vi "MakeSIGMU_Info.vi"(7 "ICM Service in":refnum<class "IcmMessageService.lvclass">, 8 "error in (no error)":errorcluster, 11 "AssetNodes In":T1[](array[typedef])) -> (0 "error out":errorcluster, 3 "SIGMU Output":T6[](array[typedef]))   [LabVIEW 2017]
uses:
  typedefs/Asset Info.ctl
  typedefs/Sensor Info.ctl
  typedefs/Metric Info.ctl
  <vilib>/addons/InsightCM/MessageBus/MessageService/IcmMessageService.lvclass
  <vilib>/addons/InsightCM/MessageBus/Base/controls/AssetNodeView.ctl
  <vilib>/addons/InsightCM/MessageBus/Base/controls/AssetState.ctl
  <vilib>/addons/InsightCM/MessageBus/Base/controls/Metric.ctl
  <vilib>/addons/InsightCM/MessageBus/Base/controls/KeyValuePair.ctl
  <vilib>/addons/InsightCM/MessageBus/Base/controls/AssetNodeReference.ctl
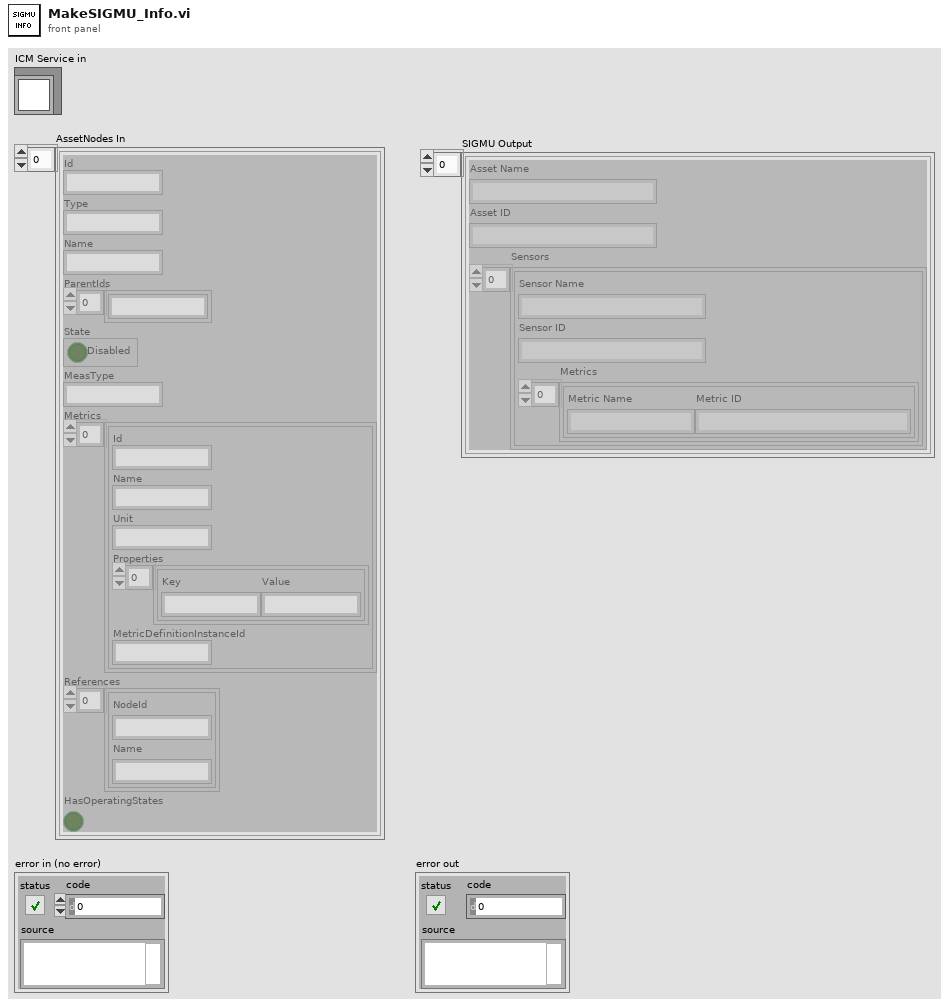
[diagram p1: front panel]
types:
  T1 = typedef "AssetNodeView.ctl" = cluster{"Id":string, "Type":string, "Name":string, "ParentIds":string[], "State":T2, "MeasType":string, "Metrics":T3[], "References":T5[], "HasOperatingStates":bool}
  T2 = typedef "AssetState.ctl" = cluster{"Disabled":bool}
  T3 = typedef "Metric.ctl" = cluster{"Id":string, "Name":string, "Unit":string, "Properties":T4[], "MetricDefinitionInstanceId":string}
  T4 = typedef "KeyValuePair.ctl" = cluster{"Key":string, "Value":string}
  T5 = typedef "AssetNodeReference.ctl" = cluster{"NodeId":string, "Name":string}
  T6 = typedef "Asset Info.ctl" = cluster{"Asset Name":string, "Asset ID":string, "Sensors":T7[]}
  T7 = typedef "Sensor Info.ctl" = cluster{"Sensor Name":string, "Sensor ID":string, "Metrics":T8[]}
  T8 = typedef "Metric Info.ctl" = cluster{"Metric Name ":string, "Metric ID":string}
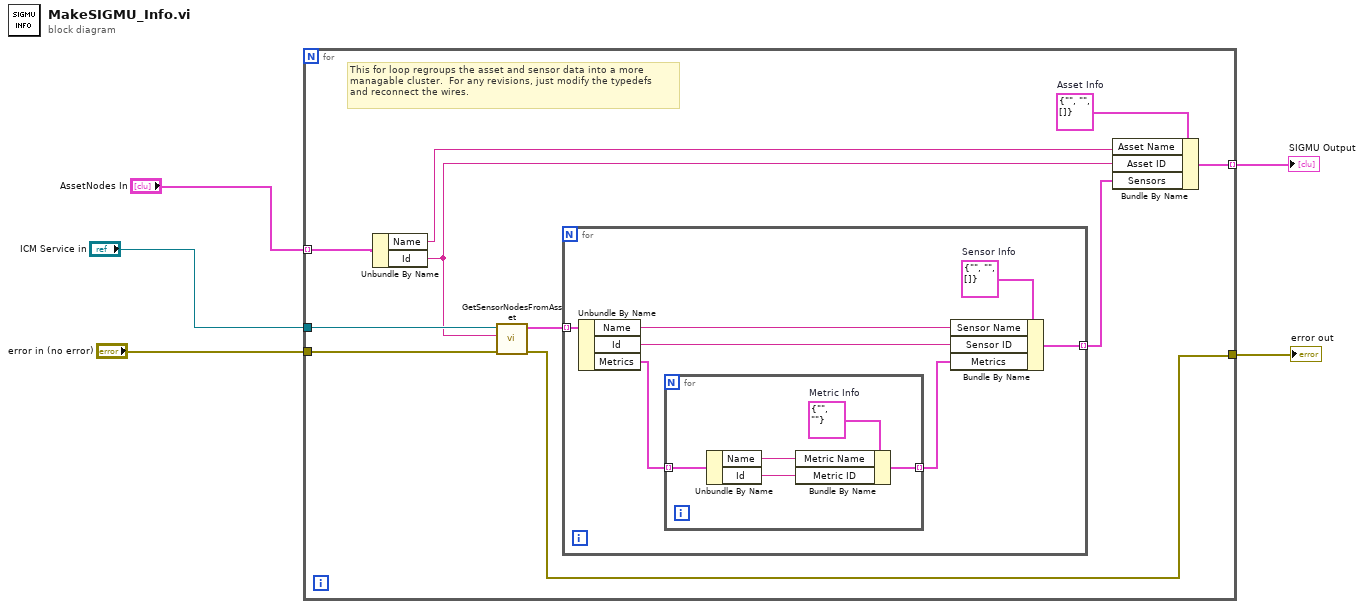
[diagram p0: block diagram]
diagram:
  n1 = for {
    tunnel: "AssetNodes In" -> [w15] mode=indexing
    tunnel: "ICM Service in" -> [w14]
    tunnel: "error in (no error)" -> [w13]
    tunnel: [w7] -> w4 mode=indexing
    tunnel: [w6] -> w5
    w12 = T6 {"Asset Name"="", "Asset ID"="", "Sensors"=[]}  # Asset Info
    # "This for loop regroups the asset and sensor data into a more \nmanagable cluster.  For any revisions, just modify the typedefs\nand reconnect the wires."
    n2 = Unbundle By Name(w15) -> ("Name"=w11:string, "Id"=w10:string)
    n3 = call "GetSensorNodesFromAsset.vi"("error in (no error)"=w13, "Asset ID"=w10, "ICM Service in"=w14) -> ("error out"=w6:errorcluster, "SensorNodes"=w9:T1[])  [unwired: 7 in]
    n4 = for {
      tunnel: w9 -> [w22] mode=indexing
      tunnel: [w16] -> w8 mode=indexing
      w21 = T7 {"Sensor Name"="", "Sensor ID"="", "Metrics"=[]}  # Sensor Info
      n5 = Unbundle By Name(w22) -> ("Name"=w20:string, "Id"=w19:string, "Metrics"=w18:T3[])
      n6 = for {
        tunnel: w18 -> [w26] mode=indexing
        tunnel: [w23] -> w17 mode=indexing
        w27 = T8 {"Metric Name "="", "Metric ID"=""}  # Metric Info
        n7 = Unbundle By Name(w26) -> ("Name"=w25:string, "Id"=w24:string)
        n8 = Bundle By Name(cluster=w27, "Metric Name"=w25, "Metric ID"=w24) -> (w23:T8)
      }
      n9 = Bundle By Name(cluster=w21, "Sensor Name"=w20, "Sensor ID"=w19, "Metrics"=w17) -> (w16:T7)
    }
    n10 = Bundle By Name(cluster=w12, "Asset Name"=w11, "Asset ID"=w10, "Sensors"=w8) -> (w7:T6)
  }
  "error out" <- w5
  "SIGMU Output" <- w4
